vi "PressureTransducerCalibration.vi"() -> ()   [LabVIEW 2021]
uses:
  <vilib>/Utility/file.llb/Write Delimited Spreadsheet (DBL).vi
panel:
  out "Recording":bool
  out "Run Time":dbl=5.0 caption="Time Target (s)"
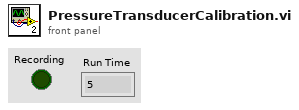
[diagram p1: front panel]
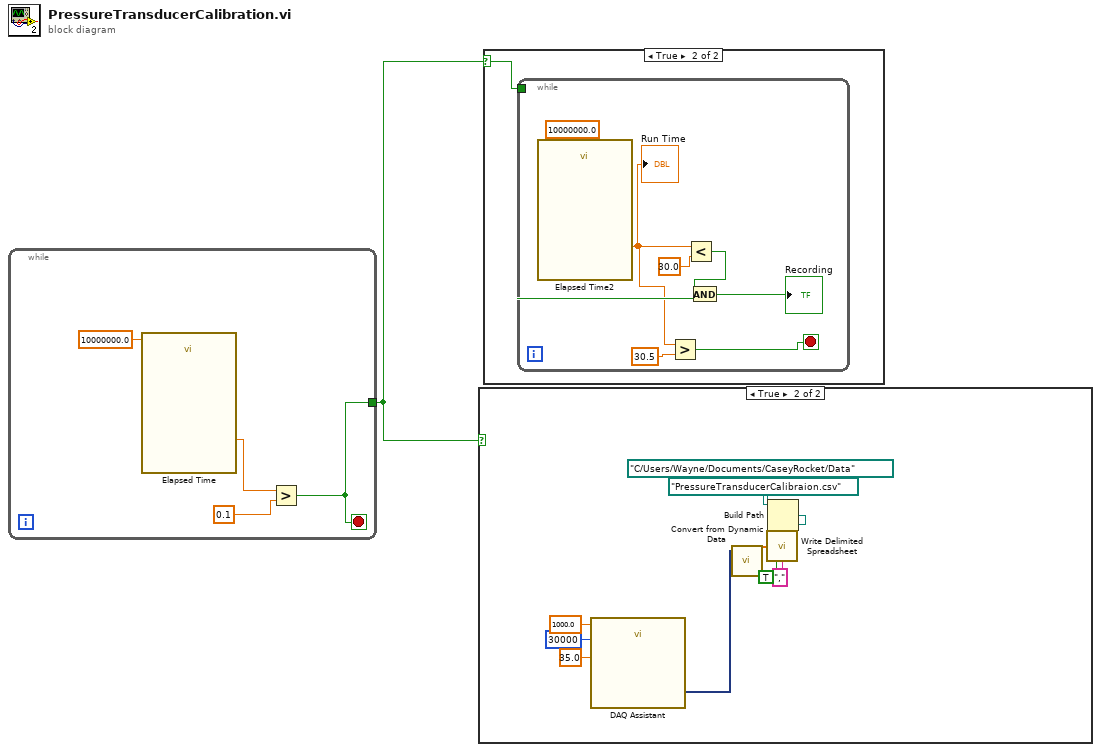
[diagram p0: block diagram]
diagram:
  n1 = while {
    tunnel: [w4] -> w1
    stop <- w4 stop-if-true
    n2 = call "Elapsed Time"("Time Target (s)"=10000000.0) -> ("Elapsed Time (s)"=w3:dbl)  [unwired: 11 in, 7 out]
    n3 = Greater?(x=w3, y=0.1) -> (0:w4:bool)
  }
  n4 = case shown="True" w1 {
    frame False {
    }
    frame True {
      n5 = call "DAQ Assistant"("rate"=1000.0, "number of samples"=30000, "timeout (s)"=35.0) -> ("data"=w6:dynamicdata)  [unwired: 14 in, 2 out]
      n6 = call "Convert from Dynamic Data"("Dynamic Data Type"=w6) -> ("Array"=w12:dbl[])  [unwired: 3 in]
      n7 = Build Path(base path=path "C:/Users/Wayne/Documents/CaseyRocket/Data", name or relative path=path "PressureTransducerCalibraion.csv") -> (appended path=w13:path)
      n8 = call-poly <vilib>:"Write Delimited Spreadsheet.vi"("file path (dialog if empty)"=w13, "1D data"=w12, "transpose? (no:F)"=TRUE, "delimiter (\\t)"="," ("delimiter (\\t)")) -> ()  [unwired: 10 in, 2 out]
    }
  }
  n9 = case shown="True" w1 {
    selector: w1 -> [_ w16]
    frame False {
    }
    frame True {
      n10 = while {
        tunnel: w16 -> [w23]
        stop <- w18 stop-if-true
        n11 = call "Elapsed Time2"("Time Target (s)"=10000000.0) -> ("Elapsed Time (s)"=w17:dbl)  [unwired: 11 in, 7 out]
        "Run Time" <- w17
        n12 = Greater?(x=w17, y=30.5) -> (0:w18:bool)
        n13 = Less?(x=w17, y=30.0) -> (x < y?=w22:bool)
        n14 = And(x=w22, y=w23) -> (x .and. y?=→"Recording":bool)
      }
    }
  }
